vi "Joysticks.vi"   [LabVIEW 2012]
uses:
  Robot Global Data.vi
  <vilib>/Rock Robotics/WPI/Joystick/WPI_JoystickGetSetRefNum.vi
types:
  T1 = typedef "WPI_JoystickDevRef.ctl" = cluster{"Device":T2}
  T2 = typedef "WPI_JoystickDeviceEnum.ctl" = enum16{"USB 1", "USB 2", "USB 3", "USB 4", "Kinect 1", "Kinect 2"}
  T3 = typedef "WPI_JoystickButtonState.ctl" = cluster{"Button 1":bool, "Button 2":bool, "Button 3":bool, "Button 4":bool, "Button 5":bool, "Button 6":bool, "Button 7":bool, "Button 8":bool, "Button 9":bool, "Button 10":bool, "Button 11":bool, "Button 12":bool}
  T4 = cluster{"axis 1 (x)":dbl, "axis 2 (y)":dbl, "axis 3 (throttle)":dbl, "axis 4":dbl, "axis 5":dbl, "axis 6":dbl}
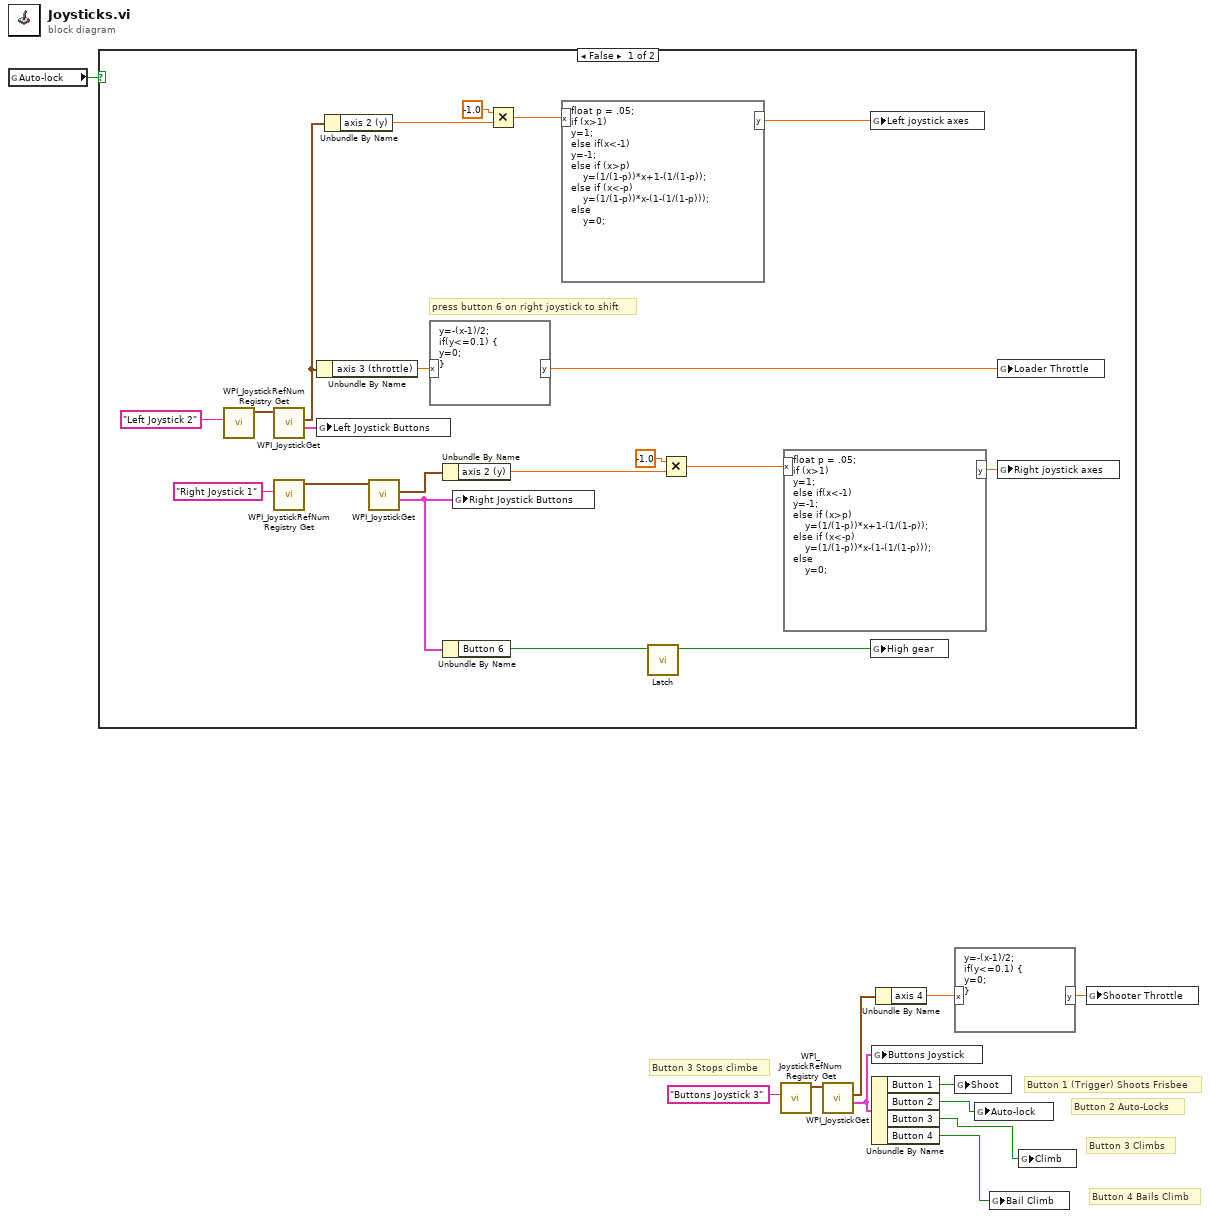
[diagram p0: block diagram]
diagram:
  # "Button 4 Bails Climb"
  # "Button 3 Climbs"
  # "Button 3 Stops climbe"
  # "Button 2 Auto-Locks"
  # "Button 1 (Trigger) Shoots Frisbee"
  n1 = global read "Robot Global Data.vi" "Auto-lock"() -> (w4:bool)
  n2 = case shown="False" w4 {
    frame False {
      # "press button 6 on right joystick to shift"
      n3 = call <vilib>:"WPI_JoystickRefNum Registry Get.vi"("refnum name"="Left Joystick 2") -> ("JoystickDevRef"=w30:T1)  [unwired: 1 in, 9 out]
      n4 = call <vilib>:"WPI_JoystickGet.vi"("JoystickDevRef"=w30) -> ("Buttons"=w25:T3, "Axes"=w13:T4)  [unwired: 1 in, 4 out]
      n5 = call <vilib>:"WPI_JoystickRefNum Registry Get.vi"("refnum name"="Right Joystick 1") -> ("JoystickDevRef"=w31:T1)  [unwired: 1 in, 9 out]
      n6 = Unbundle By Name(w13) -> ("axis 3 (throttle)"=w24:dbl)
      n7 = global write "Robot Global Data.vi" "Left Joystick Buttons"(w25) -> ()
      n8 = Unbundle By Name(w13) -> ("axis 2 (y)"=w14:dbl)
      n9 = call <vilib>:"WPI_JoystickGet.vi"("JoystickDevRef"=w31) -> ("Buttons"=w26:T3, "Axes"=w18:T4)  [unwired: 1 in, 4 out]
      n10 = formula code="y=-(x-1)/2;\nif(y<=0.1) {\ny=0;\n}"("x"=w24) -> ("y"=w23:dbl)
      n11 = Unbundle By Name(w18) -> ("axis 2 (y)"=w19:dbl)
      n12 = Unbundle By Name(w26) -> ("Button 6"=w27:bool)
      n13 = global write "Robot Global Data.vi" "Right Joystick Buttons"(w26) -> ()
      n14 = Multiply(x=-1.0, y=w14) -> (x*y=w15:dbl)
      n15 = formula code="float p = .05; \nif (x>1)\ny=1;\nelse if(x<-1)\ny=-1;\nelse if (x>p)\n    y=(1/(1-p))*x+1-(1/(1-p));\nelse if (x<-p) \n    y=(1/(1-p))*x-(1-(1/(1-p)));\nelse\n    y=0;"("x"=w15) -> ("y"=w12:dbl)
      n16 = call "Latch.vi"("Input"=w27) -> ("Output"=w28:bool)  [unwired: 9 in]
      n17 = Multiply(x=-1.0, y=w19) -> (x*y=w20:dbl)
      n18 = formula code="float p = .05; \nif (x>1)\ny=1;\nelse if(x<-1)\ny=-1;\nelse if (x>p)\n    y=(1/(1-p))*x+1-(1/(1-p));\nelse if (x<-p) \n    y=(1/(1-p))*x-(1-(1/(1-p)));\nelse\n    y=0;"("x"=w20) -> ("y"=w17:dbl)
      n19 = global write "Robot Global Data.vi" "Left joystick axes"(w12) -> ()
      n20 = global write "Robot Global Data.vi" "High gear"(w28) -> ()
      n21 = global write "Robot Global Data.vi" "Loader Throttle"(w23) -> ()
      n22 = global write "Robot Global Data.vi" "Right joystick axes"(w17) -> ()
    }
    frame True {
      # "Disables drive joystics while Auto-Lock selected"
    }
  }
  n23 = call <vilib>:"WPI_JoystickRefNum Registry Get.vi"("refnum name"="Buttons Joystick 3") -> ("JoystickDevRef"=w11:T1)  [unwired: 9 in, 1 out]
  n24 = call <vilib>:"WPI_JoystickGet.vi"("JoystickDevRef"=w11) -> ("Buttons"=w6:T3, "Axes"=w9:T4)  [unwired: 4 in, 1 out]
  n25 = global write "Robot Global Data.vi" "Buttons Joystick"(w6) -> ()
  n26 = Unbundle By Name(w6) -> ("Button 1"=w7:bool, "Button 2"=w3:bool, "Button 3"=w1:bool, "Button 4"=w2:bool)
  n27 = Unbundle By Name(w9) -> ("axis 4"=w10:dbl)
  n28 = formula code="y=-(x-1)/2;\nif(y<=0.1) {\ny=0;\n}"("x"=w10) -> ("y"=w5:dbl)
  n29 = global write "Robot Global Data.vi" "Shoot"(w7) -> ()
  n30 = global write "Robot Global Data.vi" "Auto-lock"(w3) -> ()
  n31 = global write "Robot Global Data.vi" "Bail Climb"(w2) -> ()
  n32 = global write "Robot Global Data.vi" "Climb"(w1) -> ()
  n33 = global write "Robot Global Data.vi" "Shooter Throttle"(w5) -> ()
